vi "Save GIF To File (Core).vi"(8 "error in (no error)":errorcluster, 9 "Dither (None)":T1, 10 "Image":T2, 11 "Path In":string) -> (0 "error out":errorcluster, 3 "Path Out":string)   [LabVIEW 2020, in "G-Image.lvlib"]
doc: "Saves an image in GIF format to disk."
uses:
  G-Image.lvlib
  <vilib>/picture/picture.llb/imagedata.ctl
  Controls/Dither Type.ctl
  Controls/Image Save Format.ctl
  84b65850-7e2c-4555-ae76-2c591eca4b86.vi
  Private/Debug Path.vi
  Private/Result To Error.vi
  Private/Get Image Data.vi
  Private/ARGB To RGBA.vi
  Private/Depth To Number Channels.vi
  <vilib>/Utility/file.llb/Application Directory.vi
  <vilib>/Utility/error.llb/Error Cluster From Error Code.vi
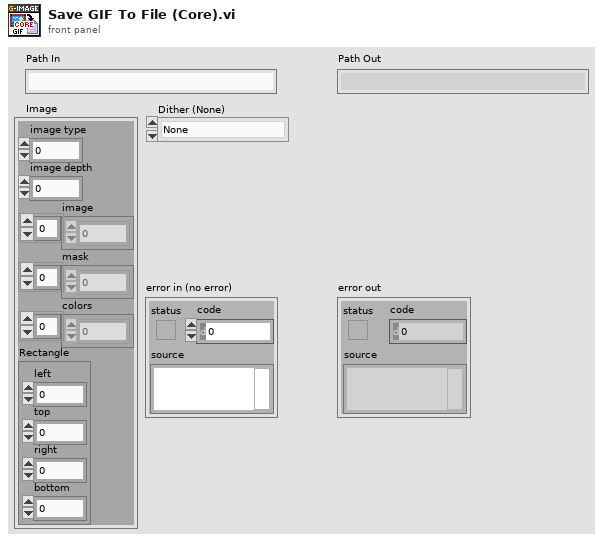
[diagram p1: front panel]
types:
  T1 = typedef "G-Image.lvlib/Dither Type.ctl" = enum32{"None", "Floyd-Steinberg"}
  T2 = typedef "imagedata.ctl" = cluster{"image type":i32, "image depth":i32, "image":u8[], "mask":u8[], "colors":u32[], "Rectangle":cluster{"left":i16, "top":i16, "right":i16, "bottom":i16}}
  T3 = typedef "G-Image.lvlib/Image Save Format.ctl" = enum16{"png", "jpg", "bmp", "gif", "tga"}
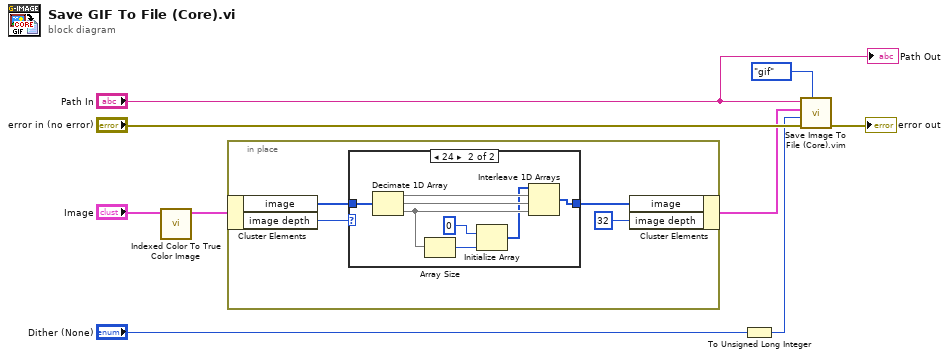
[diagram p0: block diagram]
diagram:
  n1 = call "Indexed Color To True Color Image.vi"("Indexed Image"="Image") -> ("True Color Image"=w2:T2)  [unwired: 9 in, 1 out]
  n2 = in-place {
    n3 = in-place-cluster #1(w2) -> ("image"=w12:u8[], "image depth"=w13:i32)
    n4 = case shown="24" w13 {
      tunnel: w12 -> [w14 w22]
      tunnel: [w14 w15] -> w11
      frame Default {
      }
      frame 24 {
        n5 = Decimate 1D Array(w22) -> (w21:u8[], w20:u8[], w19:u8[])
        n6 = Array Size(array=w19) -> (size(s)=w18:i32)
        n7 = Initialize Array(u8 0, w18) -> (w17:u8[])
        n8 = Interleave 1D Arrays(w17, w21, w20, w19) -> (w15:u8[])
      }
    }
    n9 = in-place-cluster #1("image"=w11, "image depth"=32) -> (w1:T2)
  }
  n10 = To Unsigned Long Integer(number="Dither (None)") -> (unsigned 32bit integer=w4:u32)
  n11 = call "Save Image To File (Core).vim"("Save Format"=Image_Save_Format."gif", "error in (no error)"="error in (no error)", "Option"=w4, "Picture"=w1, "Path In"="Path In") -> ("error out"=→"error out":errorcluster)  [unwired: 5 in, 1 out]
  "Path Out" <- "Path In"
